vi "Terminal_Friction_Torque.vi"(10 "摩擦力FR":dbl, 11 "摩擦力FL":dbl) -> (3 "摩擦力矩":dbl)   [LabVIEW 2014]
panel:
  # "摩擦力矩计算"
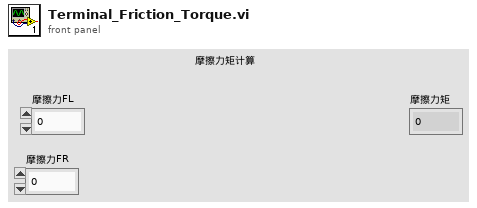
[diagram p1: front panel]
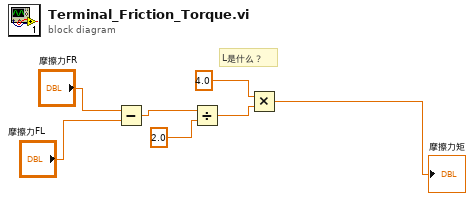
[diagram p0: block diagram]
diagram:
  # "L是什么？"
  n1 = Subtract(x="摩擦力FR", y="摩擦力FL") -> (x-y=w5:dbl)
  n2 = Divide(x=w5, y=sgl 2.0) -> (x/y=w3:dbl)
  n3 = Multiply(x=sgl 4.0, y=w3) -> (x*y=→"摩擦力矩":dbl)
